vi "Action to ActionID.vi"() -> ()   [LabVIEW 2020, in "WS Admin.lvlib"]
uses:
  WS Admin.lvlib
  WS Action.ctl
panel:
  out "Action ID":i32
  in  "Action":T1
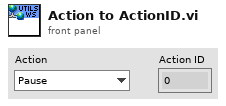
[diagram p1: front panel]
types:
  T1 = typedef "WS Admin.lvlib/WS Action.ctl" = enum16{"Pause", "Resume", "Restart", "RunState", "Unpublish"}
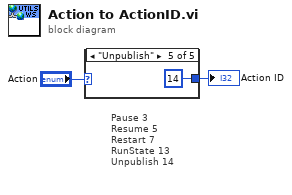
[diagram p0: block diagram]
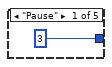
[diagram p2: hidden frame]
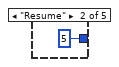
[diagram p3: hidden frame]
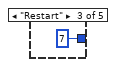
[diagram p4: hidden frame]
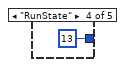
[diagram p5: hidden frame]
diagram:
  # "Pause 3\nResume 5\nRestart 7\nRunState 13\nUnpublish 14"
  n1 = case shown="\"Unpublish\"" "Action" {
    tunnel: [3 5 7 13 14] -> w1
    frame "Pause" {
    }
    frame "Resume" {
    }
    frame "Restart" {
    }
    frame "RunState" {
    }
    frame "Unpublish" {
    }
  }
  "Action ID" <- w1
